vi "MIPI_RFEE_Read Utility.vi"() -> ()   [LabVIEW 2013]
doc: "This VI demonstaits how to write to and read back data from a MIPI device. To run this VI:\n1) Change Resource name to the name of your HSDIO card\n2) The MIPI clock will run at <Sample Clock Rate>/<Oversample Factor>. This is 26 MHz (full rate). If your device should be run at a slower rate, decrease the sample clock rate and (or) increase the oversample rate.\n3. At 104MHz, the RTD value should be ~5 for a 1.5 meter cable. If you are running at a different clock rate or using a different length cable, adjust the RTD Compensation value so the MIPI data is stable at the falling edge of the clock. If you need futher timing adjustment, consider setting the data position to \"Delay from Sample Clock Rising Edge\" and configuring this delay."
uses:
  MIPI_RFFE/Ctrls/Configuration.ctl
  MIPI_RFFE/Ctrls/ClockDataChannels.ctl
  MIPI_RFFE/Ctrls/RegReadWrite.ctl
  <instrlib>/niHSDIO/niHSDIO.llb/niHSDIO_ctl Voltage Logic Family Values (Ring).ctl
  <instrlib>/niHSDIO/niHSDIO.llb/niHSDIO_ctl Sample Clock Source Values (ComboBox).ctl
  <instrlib>/niHSDIO/niHSDIO.llb/niHSDIO_ctl Data Position Values (Ring).ctl
  MIPI_RFFE/Ctrls/ExtendedRegReadWrite.ctl
  <instrlib>/niHSDIO/niHSDIO.llb/niHSDIO Configure Data Voltage Logic Family.vi
  <instrlib>/niHSDIO/niHSDIO.llb/niHSDIO Configure Digital Edge Start Trigger.vi
  <instrlib>/niHSDIO/niHSDIO.llb/niHSDIO Configure Initial State (String).vi
  <instrlib>/niHSDIO/niHSDIO.llb/niHSDIO Configure Idle State (String).vi
  <instrlib>/niHSDIO/niHSDIO.llb/niHSDIO Write Named Waveform (WDT).vi
  <instrlib>/niHSDIO/niHSDIO.llb/niHSDIO Fetch Waveform (WDT).vi
  <vilib>/Waveform/DWDTOps.llb/DWDT Append Digital Signals.vi
panel:
  in  "logic family":T1=8 items=["5.0V Logic"=5, "3.3V Logic"=6, "2.5V Logic"=7, "1.8V Logic"=8, "1.5V Logic"=80, "1.2V Logic"=81]
  in  "channel list (all:\"\")":string="2,0"
  in  "delay (0.000)":dbl format="%.3f"
  out "Parity Error":bool
  out "MIPI Data Read from DUT":cluster{"Read Data":u8[]}[](array[cluster])=[{"Read Data"=[128]}]
  in  "Register Read/Write":T2={"Slave Address"=6, "Register"=28, "Data"=0, "SetID_Pin_State"=enum."0"} {"Register" format="%.0x"; "Slave Address" max=15 format="%.0x"}
  in  "RTD Compensation Value":i32=1 min=0 max=29
  out "Digital Waveform Graph":digitalwaveform(graph)={"t0"=timestamp(3585852840.1106524 s since 1904-01-01), "dt"=5e-07, "Y"={"transitions"=[], "data"=[[1, 0, 1, 0], [1, 0, 1, 0], [1, 0, 1, 0], [1, 0, 1, 0], [1, 0, 1, 0], [1, 0, 1, 0], [1, 0, 1, 0], [1, 0, 1, 0], [0, 0, 0, 0], [0, 0, 0, 0], [0, 0, 0, 0], [0, 0, 0, 0], [0, 0, 0, 0], [0, 0, 0, 0], [0, 0, 0, 0], [0, 0, 0, 0], [0, 1, 0, 1], [0, 1, 0, 1], [0, 1, 0, 1], [0, 1, 0, 1], [0, 0, 0, 0], [0, 0, 0, 0], [0, 0, 0, 0], [0, 0, 0, 0], [1, 1, 1, 1], [1, 1, 1, 1], [1, 1, 1, 1], [1, 1, 1, 1], [1, 0, 1, 0], [1, 0, 1, 0], [1, 0, 1, 0], [1, 0, 1, 0], [1, 1, 1, 1], [1, 1, 1, 1], [1, 1, 1, 1], [1, 1, 1, 1], [1, 0, 1, 0], [1, 0, 1, 0], [1, 0, 1, 0], [1, 0, 1, 0], [0, 1, 0, 1], [0, 1, 0, 1], [0, 1, 0, 1], [0, 1, 0, 1], [0, 0, 0, 0], [0, 0, 0, 0], [0, 0, 0, 0], [0, 0, 0, 0], [0, 1, 0, 1], [0, 1, 0, 1], [0, 1, 0, 1], [0, 1, 0, 1], [0, 0, 0, 0], [0, 0, 0, 0], [0, 0, 0, 0], [0, 0, 0, 0], [1, 1, 1, 1], [1, 1, 1, 1], [1, 1, 1, 1], [1, 1, 1, 1], [1, 0, 1, 0], [1, 0, 1, 0], [1, 0, 1, 0], [1, 0, 1, 0], [0, 1, 0, 1], [0, 1, 0, 1], [0, 1, 0, 1], [0, 1, 0, 1], [0, 0, 0, 0], [0, 0, 0, 0], [0, 0, 0, 0], [0, 0, 0, 0], [1, 1, 1, 1], [1, 1, 1, 1], [1, 1, 1, 1], [1, 1, 1, 1], [1, 0, 1, 0], [1, 0, 1, 0], [1, 0, 1, 0], [1, 0, 1, 0], [1, 1, 1, 1], [1, 1, 1, 1], [1, 1, 1, 1], [1, 1, 1, 1], [1, 0, 1, 0], [1, 0, 1, 0], [1, 0, 1, 0], [1, 0, 1, 0], [1, 1, 1, 1], [1, 1, 1, 1], [1, 1, 1, 1], [1, 1, 1, 1], [1, 0, 1, 0], [1, 0, 1, 0], [1, 0, 1, 0], [1, 0, 1, 0], [0, 1, 0, 1], [0, 1, 0, 1], [0, 1, 0, 1], [0, 1, 0, 1], [0, 0, 0, 0], [0, 0, 0, 0], [0, 0, 0, 0], [0, 0, 0, 0], [0, 1, 0, 1], [0, 1, 0, 1], [0, 1, 0, 1], [0, 1, 0, 1], [0, 0, 0, 0], [0, 0, 0, 0], [0, 0, 0, 0], [0, 0, 0, 0], [1, 1, 1, 1], [1, 1, 1, 1], [1, 1, 1, 1], [1, 1, 1, 1], [1, 0, 1, 0], [1, 0, 1, 0], [1, 0, 1, 0], [1, 0, 1, 0], [1, 1, 1, 1], [1, 1, 1, 1], [1, 1, 1, 1], [1, 1, 1, 1], [1, 0, 1, 0], [1, 0, 1, 0], [1, 0, 1, 0], [1, 0, 1, 0], [0, 1, 0, 1], [0, 1, 0, 1], [0, 1, 0, 1], [0, 1, 0, 1], [0, 0, 0, 0], [0, 0, 0, 0], [0, 0, 0, 0], [0, 0, 0, 0], [0, 1, 0, 1], [0, 1, 0, 1], [0, 1, 0, 1], [0, 1, 0, 1], [0, 0, 0, 0], [0, 0, 0, 0], [0, 0, 0, 0], [0, 0, 0, 0], [0, 1, 0, 1], [0, 1, 0, 1], [0, 1, 0, 1], [0, 1, 0, 1], [0, 0, 0, 0], [0, 0, 0, 0], [0, 0, 0, 0], [0, 0, 0, 0], [0, 1, 0, 1], [0, 1, 0, 1], [0, 1, 0, 1], [0, 1, 0, 1], [0, 0, 0, 0], [0, 0, 0, 0], [0, 0, 0, 0], [0, 0, 0, 0], [0, 1, 0, 1], [0, 1, 0, 1], [0, 1, 0, 1], [0, 1, 0, 1], [0, 0, 0, 0], [0, 0, 0, 0], [0, 0, 0, 0], [0, 0, 0, 0], [0, 1, 0, 1], [0, 1, 0, 1], [0, 1, 0, 1], [0, 1, 0, 1], [0, 0, 0, 0], [0, 0, 0, 0], [0, 0, 0, 0], [0, 0, 0, 0], [0, 1, 0, 1], [0, 1, 0, 1], [0, 1, 0, 1], [0, 1, 0, 1], [0, 0, 0, 0], [0, 0, 0, 0], [0, 0, 0, 0], [0, 0, 0, 0], [0, 1, 0, 1], [0, 1, 0, 1], [0, 1, 0, 1], [0, 1, 0, 1], [0, 0, 0, 0], [0, 0, 0, 0], [0, 0, 0, 0], [0, 0, 0, 0], [0, 1, 0, 1], [0, 1, 0, 1], [0, 1, 0, 1], [0, 1, 0, 1], [0, 0, 0, 0], [0, 0, 0, 0], [0, 0, 0, 0], [0, 0, 0, 0], [1, 0, 1, 0], [1, 0, 1, 0], [1, 0, 1, 0], [1, 0, 1, 0], [1, 0, 1, 0], [1, 0, 1, 0], [1, 0, 1, 0], [1, 0, 1, 0], [0, 0, 0, 0], [0, 0, 0, 0], [0, 0, 0, 0], [0, 0, 0, 0], [0, 0, 0, 0], [0, 0, 0, 0], [0, 0, 0, 0], [0, 0, 0, 0], [0, 1, 0, 1], [0, 1, 0, 1], [0, 1, 0, 1], [0, 1, 0, 1], [0, 0, 0, 0], [0, 0, 0, 0], [0, 0, 0, 0], [0, 0, 0, 0], [1, 1, 1, 1], [1, 1, 1, 1], [1, 1, 1, 1], [1, 1, 1, 1], [1, 0, 1, 0], [1, 0, 1, 0], [1, 0, 1, 0], [1, 0, 1, 0], [1, 1, 1, 1], [1, 1, 1, 1], [1, 1, 1, 1], [1, 1, 1, 1], [1, 0, 1, 0], [1, 0, 1, 0], [1, 0, 1, 0], [1, 0, 1, 0], [0, 1, 0, 1], [0, 1, 0, 1], [0, 1, 0, 1], [0, 1, 0, 1], [0, 0, 0, 0], [0, 0, 0, 0], [0, 0, 0, 0], [0, 0, 0, 0], [0, 1, 0, 1], [0, 1, 0, 1], [0, 1, 0, 1], [0, 1, 0, 1], [0, 0, 0, 0], [0, 0, 0, 0], [0, 0, 0, 0], [0, 0, 0, 0], [1, 1, 1, 1], [1, 1, 1, 1], [1, 1, 1, 1], [1, 1, 1, 1], [1, 0, 1, 0], [1, 0, 1, 0], [1, 0, 1, 0], [1, 0, 1, 0], [1, 1, 1, 1], [1, 1, 1, 1], [1, 1, 1, 1], [1, 1, 1, 1], [1, 0, 1, 0], [1, 0, 1, 0], [1, 0, 1, 0], [1, 0, 1, 0], [1, 1, 1, 1], [1, 1, 1, 1], [1, 1, 1, 1], [1, 1, 1, 1], [1, 0, 1, 0], [1, 0, 1, 0], [1, 0, 1, 0], [1, 0, 1, 0], [1, 1, 1, 1], [1, 1, 1, 1], [1, 1, 1, 1], [1, 1, 1, 1], [1, 0, 1, 0], [1, 0, 1, 0], [1, 0, 1, 0], [1, 0, 1, 0], [1, 1, 1, 1], [1, 1, 1, 1], [1, 1, 1, 1], [1, 1, 1, 1], [1, 0, 1, 0], [1, 0, 1, 0], [1, 0, 1, 0], [1, 0, 1, 0], [0, 1, 0, 1], [0, 1, 0, 1], [0, 1, 0, 1], [0, 1, 0, 1], [0, 0, 0, 0], [0, 0, 0, 0], [0, 0, 0, 0], [0, 0, 0, 0], [0, 1, 0, 1], [0, 1, 0, 1], [0, 1, 0, 1], [0, 1, 0, 1], [0, 0, 0, 0], [0, 0, 0, 0], [0, 0, 0, 0], [0, 0, 0, 0], [0, 1, 0, 1], [0, 1, 0, 1], [0, 1, 0, 1], [0, 1, 0, 1], [0, 0, 0, 0], [0, 0, 0, 0], [0, 0, 0, 0], [0, 0, 0, 0], [0, 1, 0, 1], [0, 1, 0, 1], [0, 1, 0, 1], [0, 1, 0, 1], [0, 0, 0, 0], [0, 0, 0, 0], [0, 0, 0, 0], [0, 0, 0, 0], [1, 1, 5, 1], [1, 1, 5, 1], [1, 1, 5, 1], [1, 1, 5, 1], [1, 0, 4, 0], [1, 0, 5, 0], [1, 0, 5, 0], [1, 0, 5, 0], [0, 1, 5, 1], [0, 1, 5, 1], [0, 1, 5, 1], [0, 1, 5, 1], [0, 0, 3, 0], [0, 0, 5, 0], [0, 0, 5, 0], [0, 0, 5, 0], [0, 1, 5, 1], [0, 1, 5, 1], [0, 1, 5, 1], [0, 1, 5, 1], [0, 0, 3, 0], [0, 0, 5, 0], [0, 0, 5, 0], [0, 0, 5, 0], [0, 1, 5, 1], [0, 1, 5, 1], [0, 1, 5, 1], [0, 1, 5, 1], [0, 0, 3, 0], [0, 0, 5, 0], [0, 0, 5, 0], [0, 0, 5, 0], [0, 1, 5, 1], [0, 1, 5, 1], [0, 1, 5, 1], [0, 1, 5, 1], [0, 0, 3, 0], [0, 0, 5, 0], [0, 0, 5, 0], [0, 0, 5, 0], [0, 1, 5, 1], [0, 1, 5, 1], [0, 1, 5, 1], [0, 1, 5, 1], [0, 0, 3, 0], [0, 0, 5, 0], [0, 0, 5, 0], [0, 0, 5, 0], [0, 1, 5, 1], [0, 1, 5, 1], [0, 1, 5, 1], [0, 1, 5, 1], [0, 0, 3, 0], [0, 0, 5, 0], [0, 0, 5, 0], [0, 0, 5, 0], [0, 1, 5, 1], [0, 1, 5, 1], [0, 1, 5, 1], [0, 1, 5, 1], [0, 0, 3, 0], [0, 0, 5, 0], [0, 0, 5, 0], [0, 0, 5, 0], [0, 1, 5, 1], [0, 1, 5, 1], [0, 1, 5, 1], [0, 1, 5, 1], [0, 0, 3, 0], [0, 0, 5, 0], [0, 0, 5, 0], [0, 0, 5, 0], [0, 1, 0, 1], [0, 1, 0, 1], [0, 1, 0, 1], [0, 1, 0, 1], [0, 0, 0, 0], [0, 0, 0, 0], [0, 0, 0, 0], [0, 0, 0, 0]]}}
  in  "Configuratation":T3={"Samples to Allocate"=10000, "Oversample Factor"=1, "Clock Channel"=enum."0", "Data Channel"=enum."1"} {"Oversample Factor" min=1 max=254; "Samples to Allocate" min=1}
  out "Number of Sample Errors Read":i32
  in  "Sample Clock Rate":dbl=2000000.0 format="%#_6p"
  in  "Resource name":refnum<k15>="6556_0"
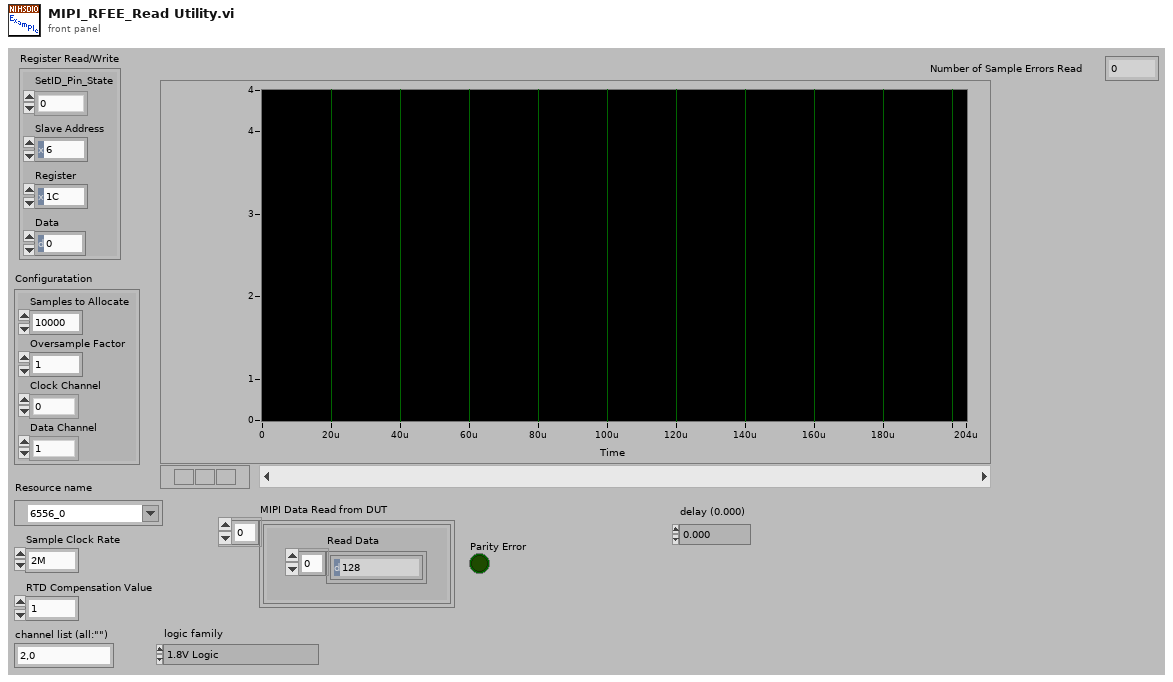
[diagram p1: front panel]
types:
  T1 = typedef "niHSDIO_ctl Voltage Logic Family Values (Ring).ctl" = i32
  T2 = typedef "RegReadWrite.ctl" = cluster{"Slave Address":u8, "Register":u8, "Data":u8, "SetID_Pin_State":enum16{"0", "1", "Z"}}
  T3 = typedef "Configuration.ctl" = cluster{"Samples to Allocate":i32, "Oversample Factor":u8, "Clock Channel":T4, "Data Channel":T4}
  T4 = typedef "ClockDataChannels.ctl" = enum16{"0", "1"}
  T5 = typedef "niHSDIO_ctl Data Position Values (Ring).ctl" = i32
  T6 = typedef "niHSDIO_ctl Sample Clock Source Values (ComboBox).ctl" = string
  T7 = typedef "RFFE_Data.ctl" = cluster{"Clock Channel":T4, "Data Channel":T4, "Oversample Factor":u8, "Zero Array":u8[], "One Array":u8[], "Z Array ":u8[], "H Array":u8[], "L Array":u8[], "X Array":u8[], "Toggle (high to low)":u8[]}
  T8 = typedef "ExtendedRegReadWrite.ctl" = cluster{"Slave Address":u8, "Register":u8, "Data":u8[]}
  T9 = typedef "ReadInfo.ctl" = cluster{"Expected Value(s)":u8[], "Compare Locations":u32[]}
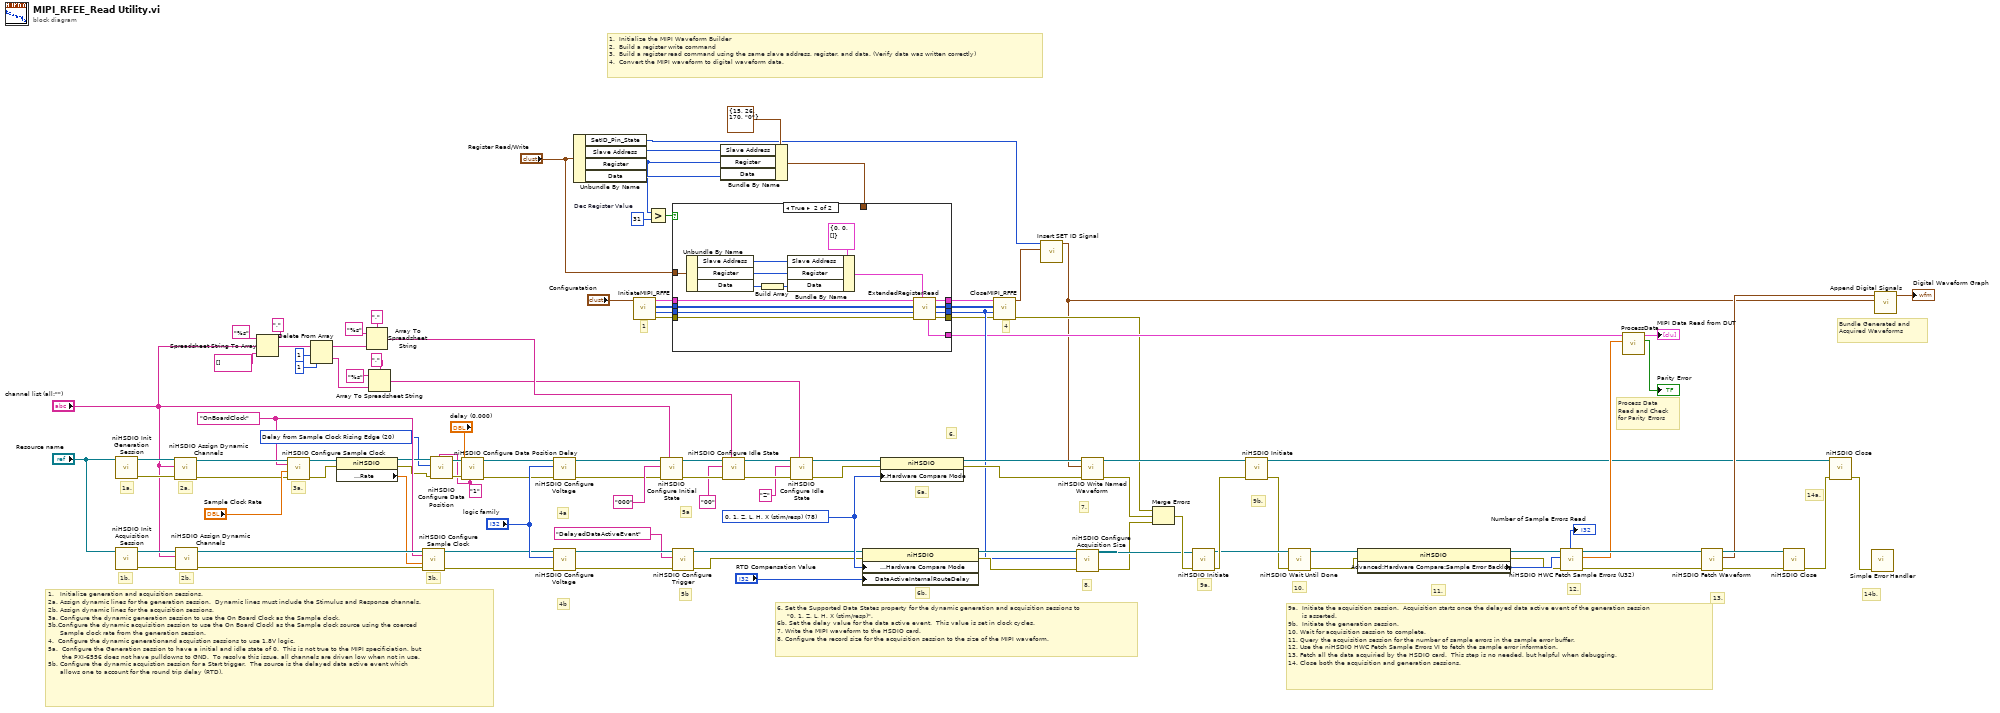
[diagram p0: block diagram]
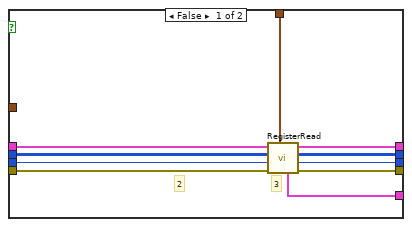
[diagram p2: hidden frame]
diagram:
  w31 = u8 31  # Dec Register Value
  w37 = T5 20 items=["Sample Clock Rising Edge"=18, "Sample Clock Falling Edge"=19, "Delay from Sample Clock Rising Edge"=20] ("position (rising edge)")
  w36 = "1" ("channel list (all:\"\")")
  w96 = 78 items=["0, 1 (binary)"=77, "0, 1, Z (tristate)"=83, "0, 1, Z, L, H, X (stim/resp)"=78, "L, H, X (resp only)"=79] ("Advanced:Supported Data States")
  w64 = T6 "OnBoardClock" ("clock source (on board clock)")
  # "4"
  # "1"
  # "1.  Initialize the MIPI Waveform Builder\n2.  Build a register write command\n3.  Build a register read command using the same slave address, register, and data. (Verify data was written correctly)\n4.  Convert the MIPI waveform to digital waveform data."
  # "Bundle Generated and Acquired Waveforms"
  # "5a"
  # "Process Data Read and Check for Parity Errors"
  # "4b"
  # "4a"
  # "13."
  # "6. Set the Supported Data States property for the dynamic generation and acquisition sessions to \n     \"0, 1, Z, L, H, X (stim/resp)\".\n6b. Set the delay value for the data active event.  This value is set in clock cycles.\n7. Write the MIPI waveform to the HSDIO card.\n8. Configure the record size for the acquisition session to the size of the MIPI waveform."
  # "6."
  # "1.   Initialize generation and acquisition sessions.\n2a. Assign dynamic lines for the generation session.  Dynamic lines must include the Stimulus and Response channels.\n2b. Assign dynamic lines for the acquisition sessions.\n3a. Configure the dynamic generation session to use the On Board Clock as the Sample clock.\n3b.Configure the dynamic acquisition session to use the On Board Clockl as the Sample clock source using the coerced \n      Sample clock rate from the generation session.\n4.  Configure the dynamic generationand acquistion sessions to use 1.8V logic.\n5a.  Configure the Generation session to have a initial and idle state of 0.  This is not true to the MIPI specificiation, but\n       the PXI-6556 does not have pulldowns to GND.  To resolve this issue, all channels are driven low when not in use.\n5b. Configure the dynamic acquistion session for a Start trigger.  The source is the delayed data active event which\n      allows one to account for the round trip delay (RTD)."
  # "14b."
  # "12."
  # "11."
  # "10."
  # "9b."
  # "9a."
  # "9a.  Initiate the acquisition session.  Acquisition starts once the delayed data active event of the generation session\n       is asserted. \n9b.  Initiate the generation session.\n10. Wait for acquisition session to complete.\n11. Query the acquisition session for the number of sample errors in the sample error buffer.\n12. Use the niHSDIO HWC Fetch Sample Errors VI to fetch the sample error information.\n13. Fetch all the data acquiried by the HSDIO card.  This step is no needed, but helpful when debugging.\n14. Close both the acquisition and generation sessions."
  # "8."
  # "7."
  # "6b."
  # "6a."
  # "5b"
  # "3b."
  # "3a."
  # "2b."
  # "2a."
  # "1b."
  # "1a."
  # "14a."
  n1 = call <instrlib>:"niHSDIO Init Generation Session.vi"("resource name"="Resource name") -> ("error out"=w67:errorcluster, "instrument handle out"=w68:refnum<k15>)  [unwired: 9 in]
  n2 = call <instrlib>:"niHSDIO Init Acquisition Session.vi"("resource name"="Resource name") -> ("error out"=w71:errorcluster, "instrument handle out"=w107:refnum<k15>)  [unwired: 9 in]
  n3 = call <instrlib>:"niHSDIO Assign Dynamic Channels.vi"("error in (no error)"=w67, "channel list (all:\"\")"="channel list (all:\"\")", "instrument handle"=w68) -> ("error out"=w94:errorcluster, "instrument handle out"=w95:refnum<k15>)  [unwired: 7 in]
  n4 = call <instrlib>:"niHSDIO Assign Dynamic Channels.vi"("error in (no error)"=w71, "channel list (all:\"\")"="channel list (all:\"\")", "instrument handle"=w107) -> ("error out"=w86:errorcluster, "instrument handle out"=w87:refnum<k15>)  [unwired: 7 in]
  n5 = Spreadsheet String To Array(delimiter (Tab)=",", format string="%s", spreadsheet string="channel list (all:\"\")", array type (2D Dbl)=string[] []) -> (array=w19:string[])
  n6 = call <instrlib>:"niHSDIO Configure Sample Clock.vi"("error in (no error)"=w94, "clock rate (50MHz)"="Sample Clock Rate", "clock source (on board clock)"=w64, "instrument handle"=w95) -> ("error out"=w65:errorcluster, "instrument handle out"=w66:refnum<k15>)  [unwired: 6 in]
  n7 = Delete From Array(array=w19, length=1, index=1) -> (deleted portion=w15:string[], array with subset deleted=w16:string[])
  n8 = property on="Property Node" class="niHSDIO"(reference=w66, error in=w65) -> (reference out=w39:refnum<k15>, error out=w38:errorcluster, "Timing:Sample Clock:Rate"=w83:dbl)
  n9 = Array To Spreadsheet String(delimiter (Tab)=",", array=w16, 3:"%s" ("format string")) -> (spreadsheet string=w3:string)
  n10 = Array To Spreadsheet String(delimiter (Tab)=",", array=w15, 3:"%s" ("format string")) -> (spreadsheet string=w1:string)
  n11 = call <instrlib>:"niHSDIO Configure Sample Clock.vi"("error in (no error)"=w86, "clock rate (50MHz)"=w83, "clock source (on board clock)"=w64, "instrument handle"=w87) -> ("error out"=w63:errorcluster, "instrument handle out"=w62:refnum<k15>)  [unwired: 6 in]
  n12 = call <instrlib>:"niHSDIO Configure Data Position.vi"("channel list (all:\"\")"=w36, "error in (no error)"=w38, "position (rising edge)"=w37, "instrument handle"=w39) -> ("error out"=w41:errorcluster, "instrument handle out"=w40:refnum<k15>)  [unwired: 6 in]
  n13 = call <instrlib>:"niHSDIO Configure Data Position Delay.vi"("channel list (all:\"\")"=w36, "error in (no error)"=w41, "delay (0.000)"="delay (0.000)", "instrument handle"=w40) -> ("error out"=w44:errorcluster, "instrument handle out"=w43:refnum<k15>)  [unwired: 6 in]
  n14 = call-poly <instrlib>:"niHSDIO Configure Voltage.vi"("error in (no error)"=w44, "logic family (3.3V logic)"="logic family", "instrument handle"=w43) -> ("error out"=w45:errorcluster, "instrument handle out"=w46:refnum<k15>)  [unwired: 7 in]
  n15 = call-poly <instrlib>:"niHSDIO Configure Voltage.vi"("error in (no error)"=w63, "logic family (3.3V logic)"="logic family", "instrument handle"=w62) -> ("error out"=w60:errorcluster, "instrument handle out"=w61:refnum<k15>)  [unwired: 7 in]
  n16 = Unbundle By Name("Register Read/Write") -> ("SetID_Pin_State"=w24:enum16{"0", "1", "Z"}, "Slave Address"=w34:u8, "Register"=w25:u8, "Data"=w30:u8)
  n17 = call "InitiateMIPI_RFFE.vi"("Configuratation In"="Configuratation") -> ("error out"=w78:errorcluster, "Number of Samples Out"=w77:i32, "Data Array"=w76:u8[][], "RFFE_Data"=w74:T7)  [unwired: 7 in]
  n18 = Greater?(x=w25, y=w31) -> (0:w29:bool)
  n19 = call-poly <instrlib>:"niHSDIO Configure Initial State.vi"("channel list"="channel list (all:\"\")", "error in (no error)"=w45, "initial state"="000" ("idle state"), "instrument handle"=w46) -> ("error out"=w48:errorcluster, "instrument handle out"=w47:refnum<k15>)  [unwired: 6 in]
  n20 = call-poly <instrlib>:"niHSDIO Configure Trigger.vi"("error in (no error)"=w60, "source (PFI 0)"="DelayedDataActiveEvent" ("channel list (all:\"\")"), "instrument handle"=w61) -> ("error out"=w56:errorcluster, "instrument handle out"=w59:refnum<k15>)  [unwired: 7 in]
  n21 = Bundle By Name(cluster=T2 {"Slave Address"=15, "Register"=26, "Data"=170, "SetID_Pin_State"=enum."0"} ("Register Read/Write"), "Slave Address"=w34, "Register"=w25, "Data"=w30) -> (w33:T2)
  n22 = case shown="True" w29 {
    tunnel: w78 -> [w112 w122]
    tunnel: w77 -> [w113 w123]
    tunnel: w76 -> [w114 w124]
    tunnel: w74 -> [w115 w125]
    tunnel: [w121 w128] -> w55
    tunnel: [w120 w129] -> w54
    tunnel: [w119 w130] -> w53
    tunnel: [w118 w131] -> w27
    tunnel: [w117 w126] -> w52
    tunnel: w33 -> [w116 _]
    tunnel: "Register Read/Write" -> [_ w136]
    frame False {
      # "3"
      # "2"
      n23 = call "RegisterRead.vi"("Register Read/Write"=w116, "error in (no error)"=w112, "Number of Samples In"=w113, "Data Array"=w114, "RFFE_Data In"=w115) -> ("error out"=w118:errorcluster, "Number of Samples Out out"=w119:i32, "Data Array Out"=w120:u8[][], "RFFE_Data Out"=w121:T7, "Compare Bits Out"=w117:T9[])  [unwired: 2 in]
    }
    frame True {
      n24 = Unbundle By Name(w136) -> ("Slave Address"=w135:u8, "Register"=w134:u8, "Data"=w133:u8)
      n25 = Build Array(w133) -> (w132:u8[])
      n26 = Bundle By Name(cluster=T8 {"Slave Address"=0, "Register"=0, "Data"=[]} ("Extended Read/Write"), "Slave Address"=w135, "Register"=w134, "Data"=w132) -> (w127:T8)
      n27 = call "ExtendedRegisterRead.vi"("Extended Read/Write"=w127, "error in (no error)"=w122, "Number of Samples In"=w123, "Data Array"=w124, "RFFE_Data In"=w125) -> ("error out"=w131:errorcluster, "Number of Samples Out out"=w130:i32, "Data Array Out"=w129:u8[][], "RFFE_Data Out"=w128:T7, "Compare Bits Out"=w126:T9[])  [unwired: 2 in]
    }
  }
  n28 = call-poly <instrlib>:"niHSDIO Configure Idle State.vi"("channel list"=w3, "error in (no error)"=w48, "idle state"="00", "instrument handle"=w47) -> ("error out"=w8:errorcluster, "instrument handle out"=w5:refnum<k15>)  [unwired: 6 in]
  n29 = call-poly <instrlib>:"niHSDIO Configure Idle State.vi"("channel list"=w1, "error in (no error)"=w8, "idle state"="Z", "instrument handle"=w5) -> ("error out"=w7:errorcluster, "instrument handle out"=w6:refnum<k15>)  [unwired: 6 in]
  n30 = property on="Property Node" class="niHSDIO"(reference=w59, error in=w56, "Advanced:Hardware Compare:Hardware Compare Mode"=w96, "DataActiveInternalRouteDelay"="RTD Compensation Value") -> (reference out=w91:refnum<k15>, error out=w90:errorcluster)
  n31 = property on="Property Node" class="niHSDIO"(reference=w6, error in=w7, "Advanced:Hardware Compare:Hardware Compare Mode"=w96) -> (reference out=w93:refnum<k15>, error out=w92:errorcluster)
  n32 = call "CloseMIPI_RFFE.vi"("error in (no error)"=w27, "Number of Samples"=w53, "Data Array"=w54, "RFFE_Data"=w55) -> ("error out"=w28:errorcluster, "Digital Waveform"=w23:digitalwaveform)  [unwired: 6 in]
  n33 = call "Insert SET ID Signal.vi"("Digital Waveform Graph"=w23, "SetID_Pin_State"=w24) -> ("Digital Waveform Graph 2"=w22:digitalwaveform)  [unwired: 9 in]
  n34 = call <instrlib>:"niHSDIO Configure Acquisition Size.vi"("error in (no error)"=w90, "samples per record (1000 samples)"=w53, "instrument handle"=w91) -> ("error out"=w85:errorcluster, "instrument handle out"=w89:refnum<k15>)  [unwired: 7 in]
  n35 = call-poly <instrlib>:"niHSDIO Write Named Waveform.vi"("error in (no error)"=w92, "data"=w22, "instrument handle"=w93) -> ("error out"=w84:errorcluster, "instrument handle out"=w98:refnum<k15>)  [unwired: 7 in]
  n36 = Merge Errors(w28, w84, w85) -> (w97:errorcluster)
  n37 = call <instrlib>:"niHSDIO Initiate.vi"("error in (no error)"=w97, "instrument handle"=w89) -> ("error out"=w106:errorcluster, "instrument handle out"=w104:refnum<k15>)  [unwired: 8 in]
  n38 = call <instrlib>:"niHSDIO Initiate.vi"("error in (no error)"=w106, "instrument handle"=w98) -> ("error out"=w102:errorcluster, "instrument handle out"=w69:refnum<k15>)  [unwired: 8 in]
  n39 = call <instrlib>:"niHSDIO Wait Until Done.vi"("error in (no error)"=w102, "instrument handle"=w104) -> ("error out"=w101:errorcluster, "instrument handle out"=w103:refnum<k15>)  [unwired: 8 in]
  n40 = property on="Property Node" class="niHSDIO"(reference=w103, error in=w101) -> (reference out=w100:refnum<k15>, error out=w99:errorcluster, "Advanced:Hardware Compare:Sample Error Backlog"=w108:i32)
  n41 = call <instrlib>:"niHSDIO HWC Fetch Sample Errors (U32).vi"("error in (no error)"=w99, "sample errors  to read"=w108, "instrument handle"=w100) -> ("error out"=w82:errorcluster, "sample numbers"=w72:dbl[], "instrument handle out"=w81:refnum<k15>, "number of sample errors read"=→"Number of Sample Errors Read":i32)  [unwired: 3 in, 2 out]
  n42 = call "ProcessData.vi"("Error Loacations"=w72, "Read Info"=w52) -> ("Parity Error"=→"Parity Error":bool, "Read MIPI Data"=→"MIPI Data Read from DUT":cluster{"Read Data":u8[]}[])  [unwired: 8 in]
  n43 = call-poly <instrlib>:"niHSDIO Fetch Waveform.vi"("error in (no error)"=w82, "instrument handle"=w81) -> ("error out"=w70:errorcluster, "data"=w75:digitalwaveform, "instrument handle out"=w110:refnum<k15>)  [unwired: 6 in, 1 out]
  n44 = call <instrlib>:"niHSDIO Close.vi"("error in (no error)"=w70, "instrument handle"=w110) -> ("error out"=w111:errorcluster)  [unwired: 9 in]
  n45 = call <instrlib>:"niHSDIO Close.vi"("error in (no error)"=w111, "instrument handle"=w69) -> ("error out"=w26:errorcluster)  [unwired: 9 in]
  n46 = call <vilib>:"Simple Error Handler.vi"("error in (no error)"=w26) -> ()  [unwired: 4 in, 5 out]
  n47 = call-poly <vilib>:"Append Digital Signals.vi"("digital waveform (low bits)"=w22, "digital waveform (high bits)"=w75) -> ("digital waveform out"=→"Digital Waveform Graph":digitalwaveform)  [unwired: 8 in, 1 out]
